vi "App Run.vi"(8 "error in (no error)":errorcluster, 11 "VolatusCoreTask in":refnum<class "VolatusCoreTask.lvclass">) -> (0 "error out":errorcluster, 3 "VolatusCoreTask out":refnum<class "VolatusCoreTask.lvclass">)   [LabVIEW 2020, in "Volatus.lvlib" / "VolatusCoreTask.lvclass"]
uses:
  VolatusCoreTask.lvclass
  VolatusCoreTask.lvclass/VolatusCoreTask.ctl
  App/App.lvclass
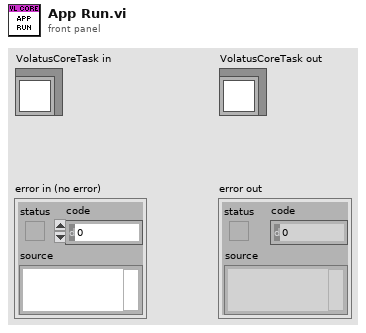
[diagram p1: front panel]
types:
  T1 = typedef "Volatus.lvlib/Core APIs.ctl" = cluster{"VolatusAPI":refnum<class "VolatusAPI.lvclass">, "EventAPI":refnum<class "EventAPI.lvclass">}
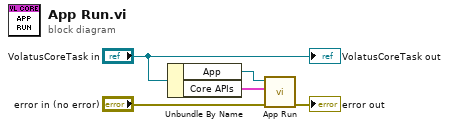
[diagram p0: block diagram]
diagram:
  n1 = Unbundle By Name("VolatusCoreTask in") -> ("App"=w2:refnum<class "App.lvclass">, "Core APIs"=w3:T1)
  n2 = call-dynamic "App Run.vi"("error in (no error)"="error in (no error)", "Core APIs"=w3, "App in"=w2) -> ("error out"=→"error out":errorcluster)  [unwired: 8 in]
  "VolatusCoreTask out" <- "VolatusCoreTask in"
